vi "NI VeriStand - Get Child Nodes.vi"(8 "Error in":errorcluster, 11 "Runtime Configuration Ref in":refnum<k39>) -> (0 "Error out":errorcluster, 2 "Child Nodes":u64[](array[numeric]), 3 "Runtime Configuration Ref out":refnum<k39>)   [LabVIEW 2027, in "Runtime Configuration File API.lvlib"]
uses:
  Runtime Configuration File API.lvlib
  C:/NetCoreDLL/NationalInstruments.VeriStand.SystemDefinitionAPI.dll
  NetCoreDLL/NationalInstruments.VeriStand.SystemDefinitionAPI.dll
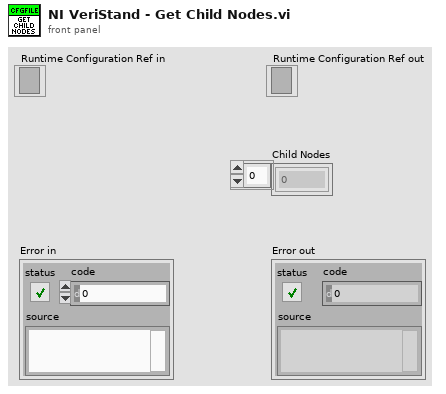
[diagram p1: front panel]
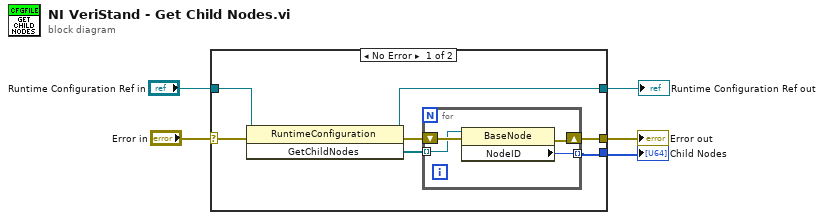
[diagram p0: block diagram]
diagram:
  n1 = case shown="No Error" "Error in" {
    selector: "Error in" -> [w12 w18]
    tunnel: "Runtime Configuration Ref in" -> [w9 w17]
    tunnel: [w8 w17] -> w2
    tunnel: [w10 w18] -> w4
    tunnel: [w6 _] -> w1
    frame No Error {
      n2 = invoke class="RuntimeConfiguration" method="GetChildNodes"(reference=w9, error in=w12) -> (reference out=w8:refnum<k39>, error out=w11:errorcluster, "GetChildNodes"=w7:refnum<k39>[])  [unwired: 1 in]
      n3 = for {
        shift-right: [w15] -> w10
        shift-left: w11 -> [w16]
        tunnel: w7 -> [w14] mode=indexing
        tunnel: [w13] -> w6 mode=indexing
        n4 = property class="BaseNode"(reference=w14, error in=w16) -> (error out=w15:errorcluster, "NodeID"=w13:u64)  [unwired: 1 out]
      }
    }
    frame Error {
    }
  }
  "Runtime Configuration Ref out" <- w2
  "Error out" <- w4
  "Child Nodes" <- w1
